vi "范围内？.vi"(10 "Coords":T2, 11 "数组":T1(array[cluster])) -> (1 "ID":string, 2 "pt in rect":bool, 3 "Index":i32)   [LabVIEW 2016]
uses:
  <vilib>/Utility/miscctls.llb/LVPoint32TypeDef.ctl
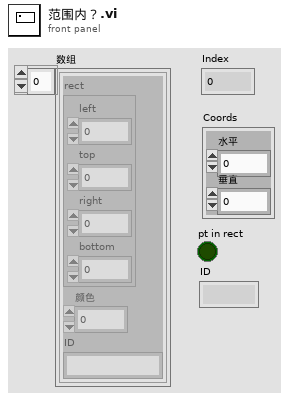
[diagram p1: front panel]
types:
  T1 = cluster{"rect":cluster{"left":i16, "top":i16, "right":i16, "bottom":i16}, "颜色":u32, "ID":string}[]
  T2 = typedef "LVPoint32TypeDef.ctl" = cluster{"Horizontal":i32, "Vertical":i32}
  T3 = cluster{"left":i16, "top":i16, "right":i16, "bottom":i16}
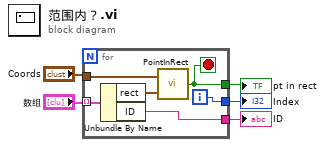
[diagram p0: block diagram]
diagram:
  n1 = for {
    tunnel: "Coords" -> [w11]
    tunnel: "数组" -> [w8] mode=indexing
    tunnel: [w10] -> w2
    tunnel: [w9] -> w5
    tunnel: [w6] -> w1
    i -> [w9]
    stop <- w10 stop-if-true
    n2 = Unbundle By Name(w8) -> ("rect"=w7:T3, "ID"=w6:string)
    n3 = call <vilib>:"PointInRect.vi"("rect"=w7, "point"=w11) -> ("pt in rect"=w10:bool)
  }
  "Index" <- w5
  "pt in rect" <- w2
  "ID" <- w1
